vi "_ConnectorPaneEditor_Interface.vi"(9 "EventsIn":T1, 10 "Events":T2) -> ()   [LabVIEW 2014, in "_ConnectorPaneEditor.lvclass"]
uses:
  _ConnectorPaneEditor.lvclass
  Pattern.ctl
  GCMCore/Providers/Veritech_GCM/Support/Framework/_Plugins/_LVCMPlugin/GCMPlugin_EventsOut.ctl
  GCMCore/Providers/Veritech_GCM/Support/Framework/_Plugins/_LVCMPlugin/GCMPlugin_EventsIn.ctl
  _ConnectorPaneEditor_States.ctl
  _ConnectorPaneEditor.lvclass/_ConnectorPaneEditor.ctl
  _ConnectorPaneEditor_Set_ vi reference.vi
  GCMCore/Providers/Veritech_GCM/Support/Framework/_Plugins/GCMPlugin/GCMPlugin.lvclass
panel:
  in  "Cancel":bool
  in  "Save":bool
  in  "CP_Picture_Ring":T3 items=["4800", "4803", "4806", "4801", "4802", "4805", "4830", "4804", "4807", "4831", "4832", "4810", "4808", "4809", "4811", "4812", "4816", "4823", "4824", "4817", "4818", "4825", "4819", "4813", "4820", "4826", "4821", "4827", "4828", "4822", "4814", "4829", "4815", "4833", "4834", "4835"]
  in  "ListOfTunels":i32(listbox)
  out "ConnectorPane":picture
  # "Warning!\nChanging pattern is irreversible operation!"
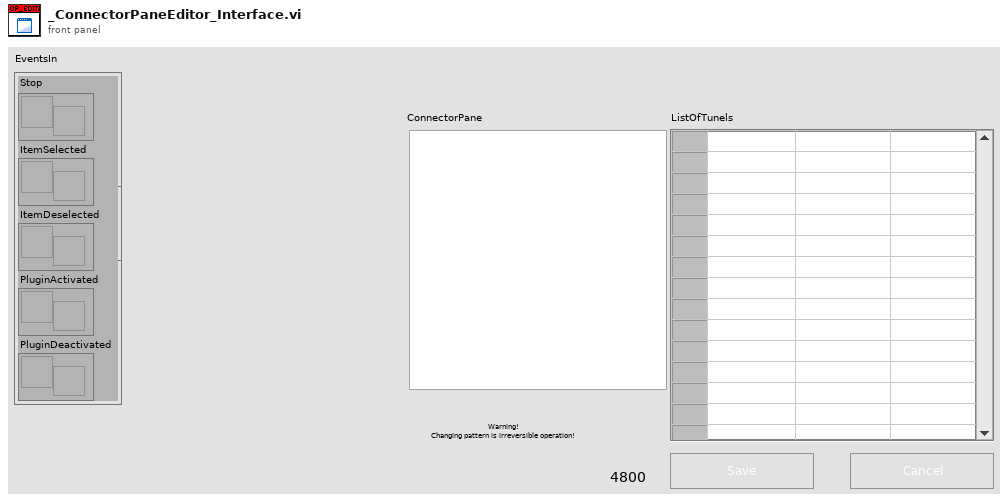
[diagram p1: front panel]
types:
  T1 = typedef "GCMPlugin.lvclass/GCMPlugin_EventsIn.ctl" = cluster{"Stop":refnum<user-event>, "ItemSelected":refnum<user-event>, "ItemDeselected":refnum<user-event>, "PluginActivated":refnum<user-event>, "PluginDeactivated":refnum<user-event>}
  T2 = typedef "GCMPlugin.lvclass/GCMPlugin_EventsOut.ctl" = cluster{"ItemEdited":refnum<user-event>}
  T3 = typedef "_ConnectorPaneEditor.lvclass/Pattern.ctl" = u16
  T4 = typedef "_ConnectorPaneEditor.lvclass/_ConnectorPaneEditor_States.ctl" = enum16{"Initialize", "SetControls", "WaitForEvent", "Save"}
  T5 = typedef "LVPoint32TypeDef.ctl" = cluster{"Horizontal":i32, "Vertical":i32}
  T6 = typedef "LVRowAndColumnTypeDef.ctl" = cluster{"Row":i32, "Column":i32}
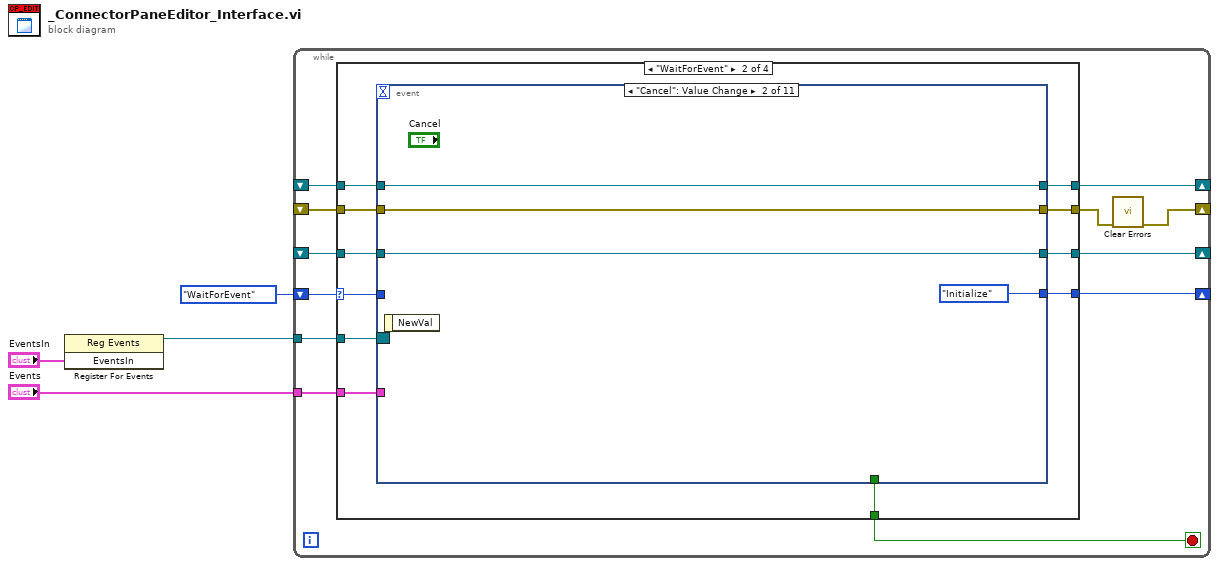
[diagram p0: block diagram]
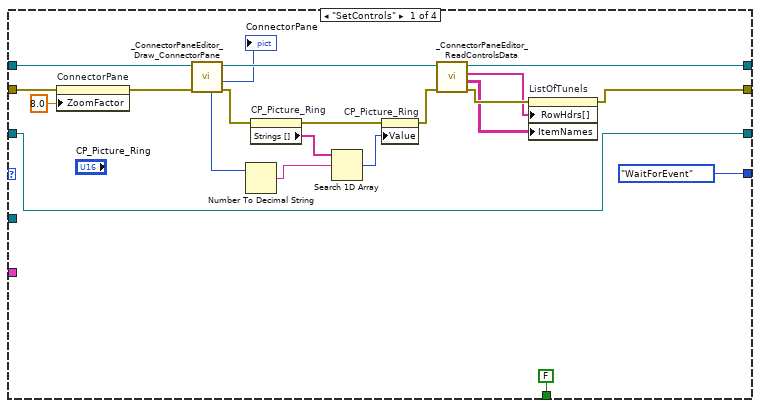
[diagram p2: hidden frame]
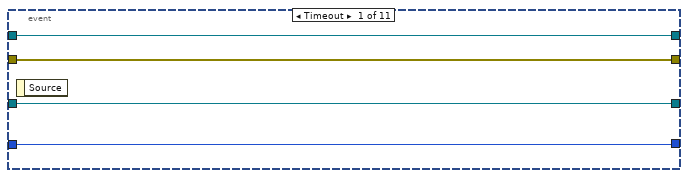
[diagram p3: hidden frame]
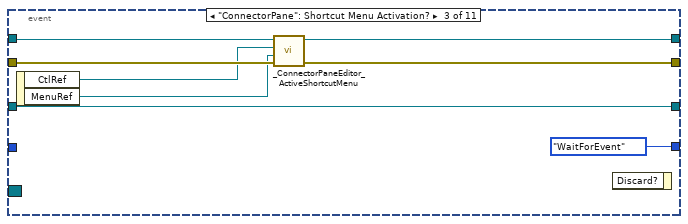
[diagram p4: hidden frame]
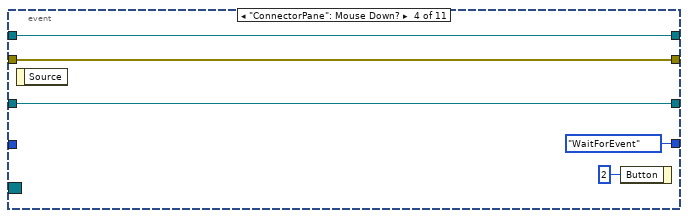
[diagram p5: hidden frame]
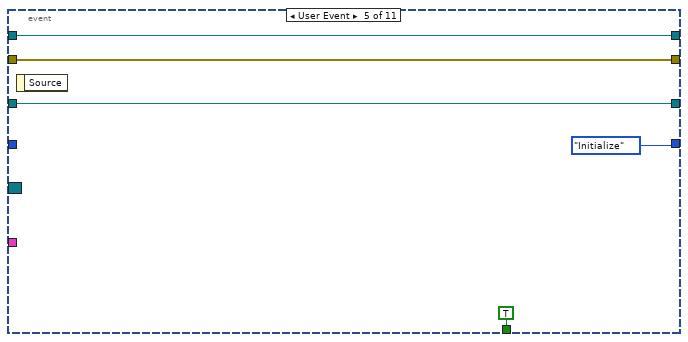
[diagram p6: hidden frame]
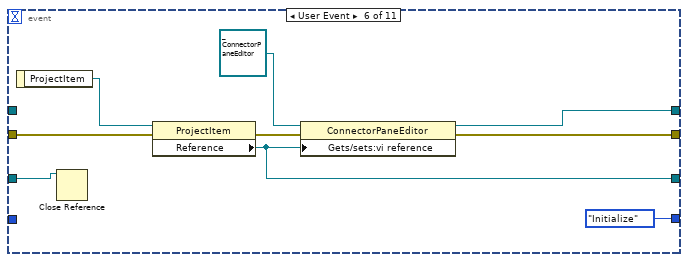
[diagram p7: hidden frame]
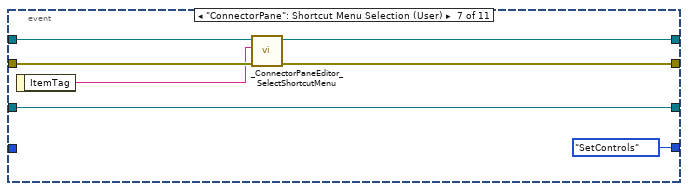
[diagram p8: hidden frame]
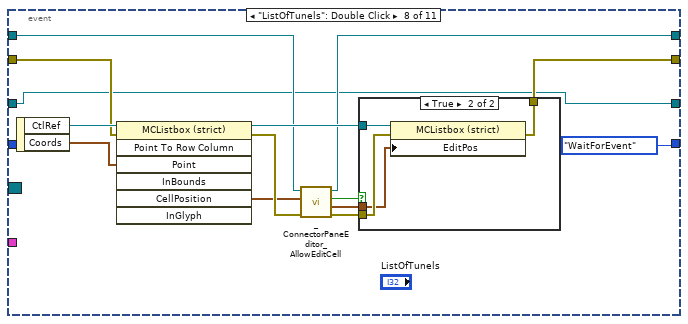
[diagram p9: hidden frame]
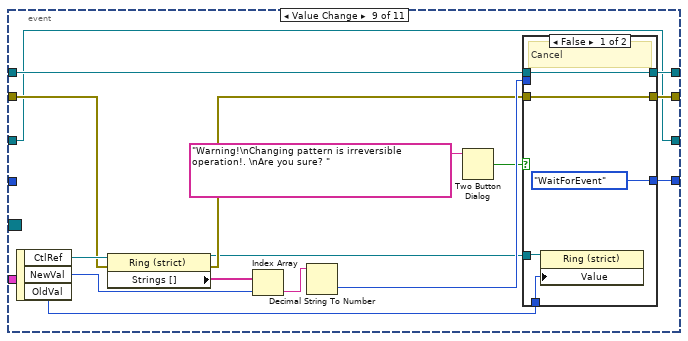
[diagram p11: hidden frame]
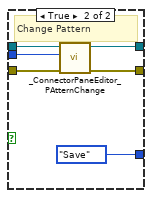
[diagram p12: hidden frame]
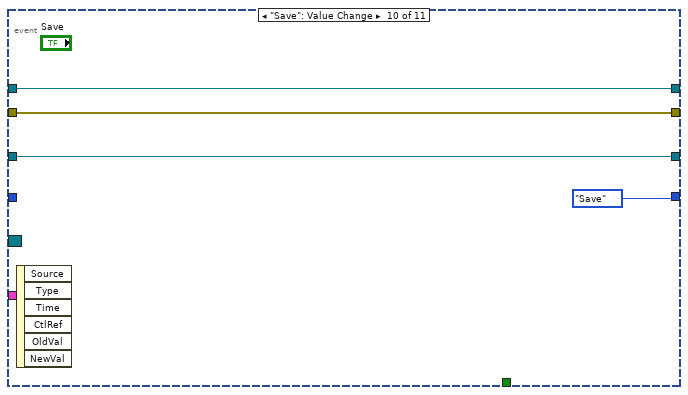
[diagram p13: hidden frame]
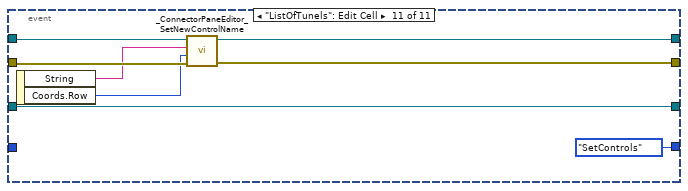
[diagram p14: hidden frame]
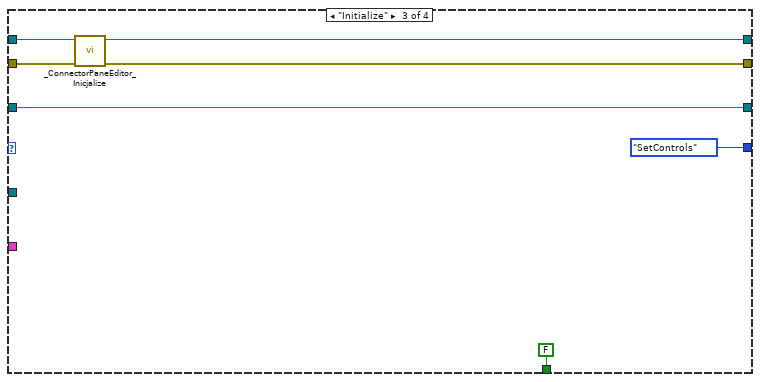
[diagram p15: hidden frame]
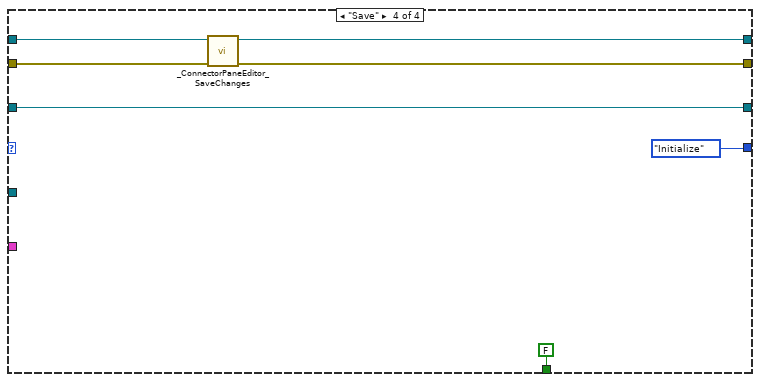
[diagram p16: hidden frame]
diagram:
  n1 = register-events("EventsIn") -> (reference out=w2:refnum<event-registration>)  [unwired: 2 in, 1 out]
  n2 = while {
    shift-right: [w12] -> _
    shift-left: _ -> [w15]
    shift-right: [w11] -> _
    shift-left: _ConnectorPaneEditor_States."WaitForEvent" -> [w16]
    tunnel: w2 -> [w9]
    tunnel: "Events" -> [w8]
    shift-right: [w6] -> _
    shift-left: _ -> [w7]
    shift-right: [w5] -> _
    shift-left: _ -> [w14]
    stop <- w10 stop-if-true
    n3 = case shown="\"WaitForEvent\"" w16 {
      selector: w16 -> [_ w42 _ _]
      tunnel: w15 -> [w31 w48 w154 w162]
      tunnel: w14 -> [w37 w47 w155 w161]
      tunnel: [w26 w44 w152 w159] -> w13
      tunnel: [w35 w43 w153 w160] -> w12
      tunnel: [_ConnectorPaneEditor_States."WaitForEvent" w45 _ConnectorPaneEditor_States."SetControls" _ConnectorPaneEditor_States."Initialize"] -> w11
      tunnel: [FALSE w46 FALSE FALSE] -> w10
      tunnel: w9 -> [_ w41 _ _]
      tunnel: w8 -> [_ w40 _ _]
      tunnel: w7 -> [w17 w39 w149 w156]
      tunnel: [w17 w38 w149 w156] -> w6
      frame "SetControls" {
        n4 = property on="ConnectorPane" class="Pict"(error in=w37, "ZoomFactor"=sgl 8.0 ("Zoom Factor")) -> (error out=w33:errorcluster)  [unwired: 1 in, 1 out]
        n5 = call "_ConnectorPaneEditor_Draw_ConnectorPane.vi"("error in (no error)"=w33, "ConnectorPaneEditor in"=w31) -> ("error out"=w24:errorcluster, "CP_Picture"=→"ConnectorPane":picture, "ConnectorPaneEditor out"=w32:refnum<class "_ConnectorPaneEditor.lvclass">, "Pattern"=w22:u32)  [unwired: 6 in]
        n6 = Number To Decimal String(number=w22) -> (decimal integer string=w21:string)  [unwired: 1 in]
        n7 = property on="CP_Picture_Ring" class="Ring (strict)"(error in=w24) -> (error out=w20:errorcluster, "Strings []"=w23:string[])  [unwired: 1 in, 1 out]
        n8 = Search 1D Array(1D array=w23, element=w21) -> (index of element=w19:i32)  [unwired: 1 in]
        n9 = property on="CP_Picture_Ring" class="Ring (strict)"(error in=w20, "Value"=w19) -> (error out=w18:errorcluster)  [unwired: 1 in, 1 out]
        n10 = call "_ConnectorPaneEditor_ReadControlsData.vi"("error in (no error)"=w18, "ConnectorPaneEditor in"=w32) -> ("error out"=w29:errorcluster, "TunelsInformation"=w27:string[][], "RowHeader"=w28:string[], "ConnectorPaneEditor out"=w35:refnum<class "_ConnectorPaneEditor.lvclass">)  [unwired: 6 in]
        n11 = property on="ListOfTunels" class="MCListbox (strict)"(error in=w29, "RowHdrs[]"=w28, "ItemNames"=w27) -> (error out=w26:errorcluster)  [unwired: 1 in, 1 out]
      }
      frame "WaitForEvent" {
        n12 = event shown="[1] \"Cancel\": Value Change" {
          selector: w41 -> [_ _ _ _ _ _ _ _ _ _ _]
          dyn-events: _ -> [_ _ _ _ _ _ _ _ _ _ _]
          timeout: _ -> [_ _ _ _ _ _ _ _ _ _ _]
          tunnel: w48 -> [w51 w54 w64 w67 w74 _ w90 w98 w125 w140 w147]
          tunnel: w47 -> [w52 w55 w63 w68 w73 w76 w89 w100 w116 w139 w146]
          tunnel: [_ _ _ _ TRUE _ _ _ _ _ _] -> w46
          tunnel: [w50 _ConnectorPaneEditor_States."Initialize" _ConnectorPaneEditor_States."WaitForEvent" _ConnectorPaneEditor_States."WaitForEvent" _ConnectorPaneEditor_States."Initialize" _ConnectorPaneEditor_States."Initialize" _ConnectorPaneEditor_States."SetControls" _ConnectorPaneEditor_States."WaitForEvent" w122 _ConnectorPaneEditor_States."Save" _ConnectorPaneEditor_States."SetControls"] -> w45
          tunnel: [w52 w55 w60 w68 w73 w78 w86 w99 w123 w139 w142] -> w44
          tunnel: [w51 w54 w61 w67 w74 w77 w87 w97 w124 w140 w143] -> w43
          tunnel: w42 -> [w50 _ _ _ _ _ _ _ _ _ _]
          tunnel: w40 -> [_ _ _ _ _ _ _ _ _ _ _]
          tunnel: w39 -> [w49 w53 w57 w65 w70 w75 w84 w91 w110 w137 w141]
          tunnel: [w49 w53 w57 w65 w70 w80 w84 w91 w110 w137 w141] -> w38
          event Timeout {
            n13 = event-data() -> ()  [unwired: 1 in, 1 out]
          }
          event "Cancel": Value Change {
            n14 = event-data() -> ()  [unwired: 1 in, 1 out]
          }
          event "ConnectorPane": Shortcut Menu Activation? {
            n15 = event-data() -> ("CtlRef"=w62:refnum<vi>, "MenuRef"=w58:refnum<k9>)  [unwired: 1 in]
            n16 = call "_ConnectorPaneEditor_ActiveShortcutMenu.vi"("error in (no error)"=w63, "MenuRef"=w58, "CPpictureRef"=w62, "ConnectorPaneEditor in"=w64) -> ("error out"=w60:errorcluster, "ConnectorPaneEditor out"=w61:refnum<class "_ConnectorPaneEditor.lvclass">)  [unwired: 6 in]
            n17 = event-data() -> ()  [unwired: 2 in, 1 out]
          }
          event "ConnectorPane": Mouse Down? {
            n18 = event-data() -> ()  [unwired: 1 in, 1 out]
            n19 = event-data("Button"=u16 2) -> ()  [unwired: 1 in, 1 out]
          }
          event User Event {
            n20 = event-data() -> ()  [unwired: 1 in, 1 out]
          }
          event User Event {
            n21 = event-data() -> ("ProjectItem"=w81:refnum<vi>)  [unwired: 1 in]
            n22 = Close Reference(reference=w75) -> ()  [unwired: 1 in, 1 out]
            n23 = property class="ProjectItem"(reference=w81, error in=w76) -> (error out=w83:errorcluster, "Reference"=w80:refnum<vi>)  [unwired: 1 out]
            n24 = property class="ConnectorPaneEditor"(reference=refnum<class "_ConnectorPaneEditor.lvclass"> refnum ("ConnectorPaneEditor.lvclass"), error in=w83, "Gets/sets:vi reference"=w80) -> (reference out=w77:refnum<class "_ConnectorPaneEditor.lvclass">, error out=w78:errorcluster)
          }
          event "ConnectorPane": Shortcut Menu Selection (User) {
            n25 = event-data() -> ("ItemTag"=w88:string)  [unwired: 1 in]
            n26 = call "_ConnectorPaneEditor_SelectShortcutMenu.vi"("error in (no error)"=w89, "ItemTag"=w88, "ConnectorPaneEditor in"=w90) -> ("error out"=w86:errorcluster, "ConnectorPaneEditor out"=w87:refnum<class "_ConnectorPaneEditor.lvclass">)  [unwired: 7 in]
          }
          event "ListOfTunels": Double Click {
            n27 = event-data() -> ("CtlRef"=w103:refnum<vi>, "Coords"=w104:T5)  [unwired: 1 in]
            n28 = invoke on="Invoke Node" class="MCListbox (strict)" method="Point To Row Column"(reference=w103, error in=w100, "Point"=w104) -> (reference out=w101:refnum<vi>, error out=w96:errorcluster, "CellPosition"=w95:T6)  [unwired: 4 in, 4 out]
            n29 = call "_ConnectorPaneEditor_AllowEditCell.vi"("error in (no error)"=w96, "Cell Position"=w95, "ConnectorPaneEditor in"=w98) -> ("error out"=w94:errorcluster, "EditPos"=w93:T6, "Allow?"=w92:bool, "ConnectorPaneEditor out"=w97:refnum<class "_ConnectorPaneEditor.lvclass">)  [unwired: 5 in]
            n30 = case shown="True" w92 {
              tunnel: w101 -> [_ w109]
              tunnel: [w105 w108] -> w99
              tunnel: w94 -> [w105 w107]
              tunnel: w93 -> [_ w106]
              frame False {
              }
              frame True {
                n31 = property class="MCListbox (strict)"(reference=w109, error in=w107, "EditPos"=w106) -> (error out=w108:errorcluster)  [unwired: 1 out]
              }
            }
          }
          event Value Change {
            n32 = event-data() -> ("CtlRef"=w121:refnum<vi>, "NewVal"=w119:T3, "OldVal"=w111:T3)  [unwired: 1 in]
            n33 = property class="Ring (strict)"(reference=w121, error in=w116) -> (reference out=w112:refnum<vi>, error out=w115:errorcluster, "Strings []"=w120:string[])
            n34 = Index Array(array=w120, index=w119) -> (element=w118:string)
            n35 = Decimal String To Number(string=w118) -> (number=w117:i32)  [unwired: 2 in, 1 out]
            n36 = Two Button Dialog(message="Warning!\nChanging pattern is irreversible operation!. \nAre you sure? ") -> (T button?=w114:bool)  [unwired: 2 in]
            n37 = case shown="False" w114 {
              tunnel: w125 -> [w130 w136]
              tunnel: [w130 w135] -> w124
              tunnel: [w129 w134] -> w123
              tunnel: [_ConnectorPaneEditor_States."WaitForEvent" _ConnectorPaneEditor_States."Save"] -> w122
              tunnel: w117 -> [_ w132]
              tunnel: w115 -> [w129 w131]
              tunnel: w112 -> [w127 _]
              tunnel: w111 -> [w126 _]
              frame False {
                # "Cancel"
                n38 = property class="Ring (strict)"(reference=w127, "Value"=w126) -> ()  [unwired: 1 in, 2 out]
              }
              frame True {
                # "Change Pattern"
                n39 = call "_ConnectorPaneEditor_PAtternChange.vi"("error in (no error)"=w131, "NewVal"=w132, "ConnectorPaneEditor in"=w136) -> ("error out"=w134:errorcluster, "ConnectorPaneEditor out"=w135:refnum<class "_ConnectorPaneEditor.lvclass">)  [unwired: 7 in]
              }
            }
          }
          event "Save": Value Change {
            n40 = event-data() -> ()  [unwired: 1 in, 6 out]
          }
          event "ListOfTunels": Edit Cell {
            n41 = event-data() -> ("String"=w145:string, "Coords.Row"=w144:i32)  [unwired: 1 in]
            n42 = call "_ConnectorPaneEditor_SetNewControlName.vi"("error in (no error)"=w146, "Row"=w144, "NewString"=w145, "ConnectorPaneEditor in"=w147) -> ("error out"=w142:errorcluster, "ConnectorPaneEditor out"=w143:refnum<class "_ConnectorPaneEditor.lvclass">)  [unwired: 6 in]
          }
        }
      }
      frame "Initialize" {
        n43 = call "_ConnectorPaneEditor_Inicjalize.vi"("error in (no error)"=w155, "ConnectorPaneEditor in"=w154) -> ("error out"=w152:errorcluster, "ConnectorPaneEditor out"=w153:refnum<class "_ConnectorPaneEditor.lvclass">)  [unwired: 8 in]
      }
      frame "Save" {
        n44 = call "_ConnectorPaneEditor_SaveChanges.vi"("error in (no error)"=w161, "ConnectorPaneEditor in"=w162) -> ("error out"=w159:errorcluster, "ConnectorPaneEditor out"=w160:refnum<class "_ConnectorPaneEditor.lvclass">)  [unwired: 8 in]
      }
    }
    n45 = call <vilib>:"Clear Errors.vi"("error in (no error)"=w13) -> ("error out"=w5:errorcluster)  [unwired: 5 in, 1 out]
  }
